vi "arduinoShakeServo.vi"(0 "shakeSpan":i8 max=63 step=1, 1 "servo position":u16(knob)=260 max=2500 step=1 scale=260.0..1150.0, 2 "channel":u8 max=15 step=1) -> ()   [LabVIEW 2012]
uses:
  GlobalArduino.vi
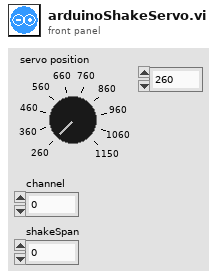
[diagram p1: front panel]
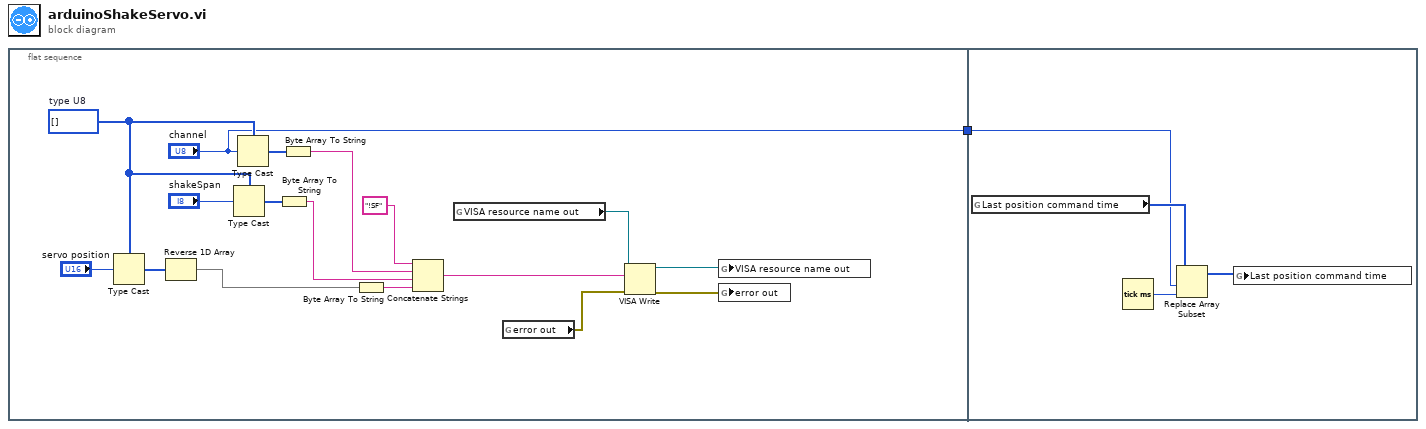
[diagram p0: block diagram]
diagram:
  n1 = flat-sequence {
    tunnel: ["channel"] -> w1
    tunnel: w1 -> [w19]
    frame #0 {
      w12 = u8[] []  # type U8
      n2 = Type Cast(type=w12, x="servo position") -> (*(type *) &x=w15:u8[])
      n3 = Reverse 1D Array(array=w15) -> (reversed array=w8:u8[])
      n4 = Type Cast(type=w12, x="shakeSpan") -> (*(type *) &x=w11:u8[])
      n5 = Type Cast(type=w12, x="channel") -> (*(type *) &x=w13:u8[])
      n6 = Byte Array To String(unsigned byte array=w11) -> (string=w10:string)
      n7 = Byte Array To String(unsigned byte array=w13) -> (string=w14:string)
      n8 = Byte Array To String(unsigned byte array=w8) -> (string=w16:string)
      n9 = Concatenate Strings("!SF" ("string"), w14, w10, w16) -> (w7:string)
      n10 = global read "GlobalArduino.vi" "VISA resource name out"() -> (w6:refnum<visa-resource-name>)
      n11 = global read "GlobalArduino.vi" "error out"() -> (w4:errorcluster)
      n12 = VISA Write(VISA resource name=w6, write buffer=w7, error in (no error)=w4) -> (VISA resource name out=w5:refnum<visa-resource-name>, error out=w3:errorcluster)  [unwired: 1 out]
      n13 = global write "GlobalArduino.vi" "VISA resource name out"(w5) -> ()
      n14 = global write "GlobalArduino.vi" "error out"(w3) -> ()
    }
    frame #1 {
      n15 = global read "GlobalArduino.vi" "Last position command time"() -> (w21:u64[])
      n16 = Tick Count (ms)() -> (millisecond timer value=w20:u32)
      n17 = Replace Array Subset(array=w21, new element=w20, index=w19) -> (w22:u64[])
      n18 = global write "GlobalArduino.vi" "Last position command time"(w22) -> ()
    }
  }
